vi "Usage Example.vi"() -> ()   [LabVIEW 2017, in "Client.lvlib" / "ParserSorter.lvlib"]
uses:
  ParserSorter.lvlib
  <vilib>/addons/database/Auxilliary.llb/DB Tools DataTypes.ctl
  SR Data.ctl
  AE Group.ctl
  SR Status.ctl
  SR Level.ctl
  SR Type.ctl
  <vilib>/addons/database/Connection.llb/DB Tools Open Connec (String).vi
  <vilib>/addons/database/NI_Database_API.lvlib
panel:
  out "Assigned":T1[](array[typedef])
  out "error out":errorcluster
  out "Unassigned":T1[](array[typedef])
  out "columns":string[](array[string])=["SR_NUMBER", "AE_GROUP", "SR_OWNER", "SR_SUMMARY", "SR_LAST_UPDATE_DATE", "FIRST_NAME", "LAST_NAME", "COMPANY", "SR_CREATION_DATE", "SR_TYPE", "SR_STATUS", "SERVICE_LEVEL", "CHANNEL", "DAYS_OPEN"]
  out "column information":T7(array[cluster])=[{"name"="SR_NUMBER", "database data type"=enum."String", "defined size"=64}, {"name"="AE_GROUP", "database data type"=enum."String", "defined size"=60}, {"name"="SR_OWNER", "database data type"=enum."String", "defined size"=721}, {"name"="SR_SUMMARY", "database data type"=enum."String", "defined size"=240}, {"name"="SR_LAST_UPDATE_DATE", "database data type"=enum."Date/Time", "defined size"=16}, {"name"="FIRST_NAME", "database data type"=enum."String", "defined size"=150}, {"name"="LAST_NAME", "database data type"=enum."String", "defined size"=150}, {"name"="COMPANY", "database data type"=enum."String", "defined size"=360}, {"name"="SR_CREATION_DATE", "database data type"=enum."Date/Time", "defined size"=16}, {"name"="SR_TYPE", "database data type"=enum."String", "defined size"=90}, {"name"="SR_STATUS", "database data type"=enum."String", "defined size"=90}, {"name"="SERVICE_LEVEL", "database data type"=enum."String", "defined size"=150}, {"name"="CHANNEL", "database data type"=enum."String", "defined size"=50}, {"name"="DAYS_OPEN", "database data type"=enum."Double (DBL)", "defined size"=8}]
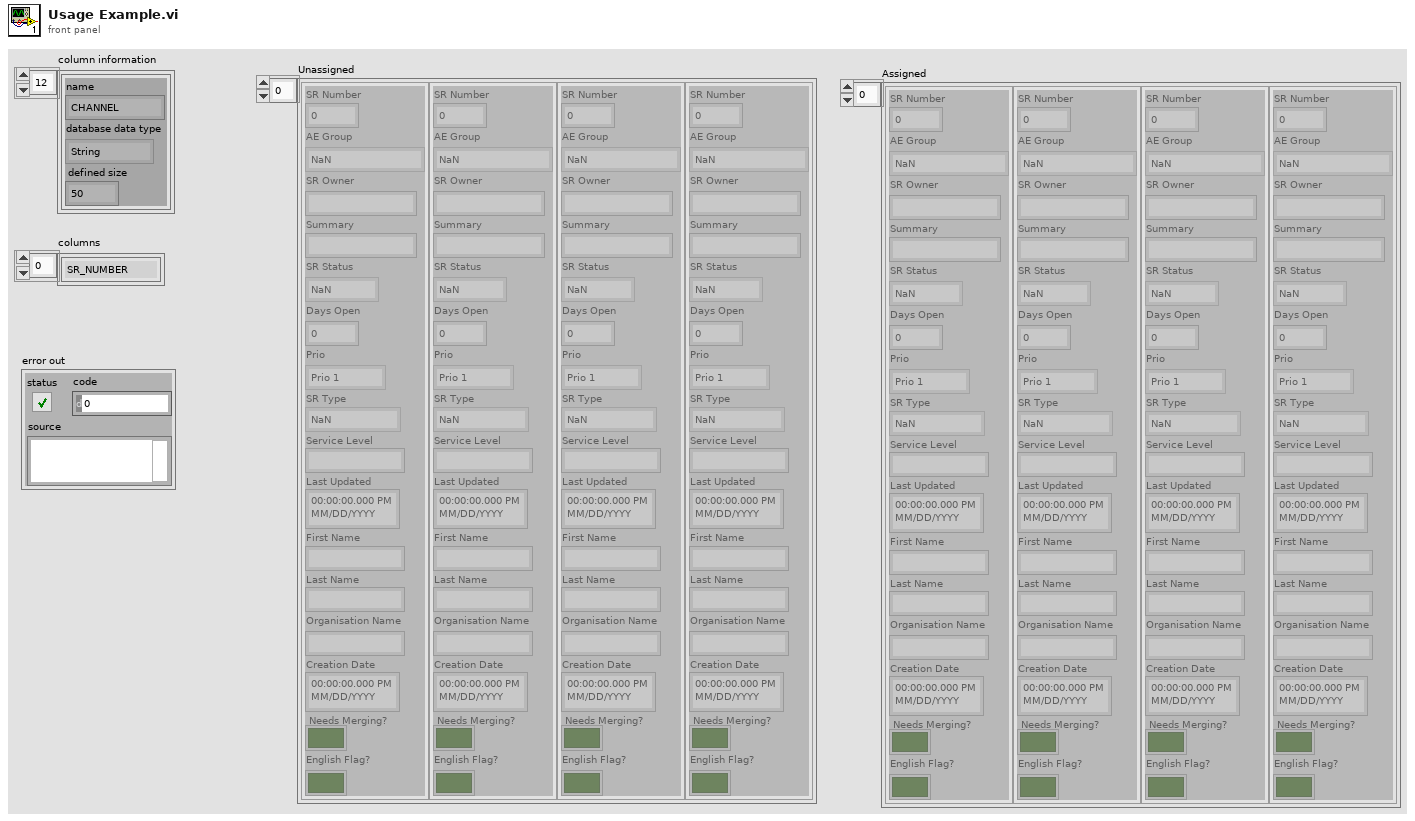
[diagram p1: front panel]
types:
  T1 = typedef "Client.lvlib/ParserSorter.lvlib/SR Data.ctl" = cluster{"SR Number":i64, "AE Group":T2, "SR Owner":string, "Summary":string, "SR Status":T3, "Days Open":dbl, "Prio":T4, "SR Type":T5, "Service Level":string, "Last Updated":timestamp, "First Name":string, "Last Name":string, "Organisation Name":string, "Creation Date":timestamp, "Needs Merging?":bool, "English Flag?":bool}
  T2 = typedef "Client.lvlib/ParserSorter.lvlib/AE Group.ctl" = enum32{"NaN", "AE-Germany", "AE-Poland", "AE-Switzerland", "AE-Czech Republic", "AE-Hungary", "AE-Romania", "AE-Slovakia", "AE-Slovenia"}
  T3 = typedef "Client.lvlib/ParserSorter.lvlib/SR Status.ctl" = enum32{"NaN", "Caller Abandoned", "Created in Error", "Declined to Purchase Support", "Expired", "Forum Resolved AE", "Forum Resolved Customer", "IN WORK", "IN WORK Collab with AES", "IN WORK Collab with PSE", "IN WORK Collab with SE", "IN WORK Escalation", "IN WORK Customer Added Note", "Open", "Potentially Resolved", "POC Resolved", "Resolved", "RMA Waiting on Customer", "RMA Open", "RMA In Progress", "RMA Closed - DOA", "RMA Closed", "RMA Approved for Return", "Project Complete", "Presumed Resolved", "IN WORK Wait on Customer"}
  T4 = typedef "Client.lvlib/ParserSorter.lvlib/SR Level.ctl" = enum16{"Prio 1", "Prio 2", "Prio 3", "Prio 4"}
  T5 = typedef "Client.lvlib/ParserSorter.lvlib/SR Type.ctl" = enum32{"NaN", "ATE Core Configurations (BYOATE)", "Activation", "BioBench", "CAN", "CM C Series", "Calibration", "Consulting Services", "CounterTimer", "DAQExpress", "DASYLab", "DIAdem", "DMM", "DSA HW", "Digital_IO", "FIRST (NIC Only)", "FieldBus", "FieldPoint", "Functional Savety", "GATI", "GPIB", "HMI and Industrial PCs", "HiQ", "HighSpeedDigital_IO", "IMAQ", "IOTech Vibration", "Industrial Communications", "InsightCM", "LV", "LV CD&Sim", "LV Comms", "LV Controls Add-Ons", "LV Embedded", "LV MathScript RT", "LV NXG", "LV NXT", "LVDSC", "LVFPGA", "LVPDA and LV Touch Panel", "LVRT", "LabWindows_CVI", "Lookout", "MATRIXx", "MStudioDotNet", "MStudioVisualBasic", "MStudioVisualC", "Measure (Legacy)", "Motion", "MultifunctionDAQ", "Multimedia Test HW/SW", "Multisim (EWB)", "NI Update Service", "OPC Servers", "Optical (OSI)", "PXI Controllers, Chassis, MXI", "PXI Timing and Sync", "Power Supplies and SMUs", "Powertrain Controls", "RAID", "RF", "RF Software", "RIO", "SC Express", "SCC", "SCXI", "SPEEDY-33 (Hyperception)", "STS", "ScopeDigitizers", "Serial", "Signal Sources", "SignalCondOther", "SignalExpress", "Software Defined Intruments", "Sound and Vibration SW", "Switch Executive", "Switches", "TestStand", "USRP", "Ultiboard (EWB)", "VBench", "VI Logger", "VXI_MXI", "VeriStand", "VisionSW", "VolumeLicenseMgr", "WSN", "Web UI Builder", "myRIO"}
  T6 = typedef "NI_Database_API.lvlib/DB Tools DataTypes.ctl" = enum16{"String", "Long (I32)", "Single (SGL)", "Double (DBL)", "Date/Time", "Binary"}
  T7 = cluster{"name":string, "database data type":T6, "defined size":i32}[]
  T8 = typedef "NI_Database_API.lvlib/Conn ObjectReference.ctl" = refnum<k1>
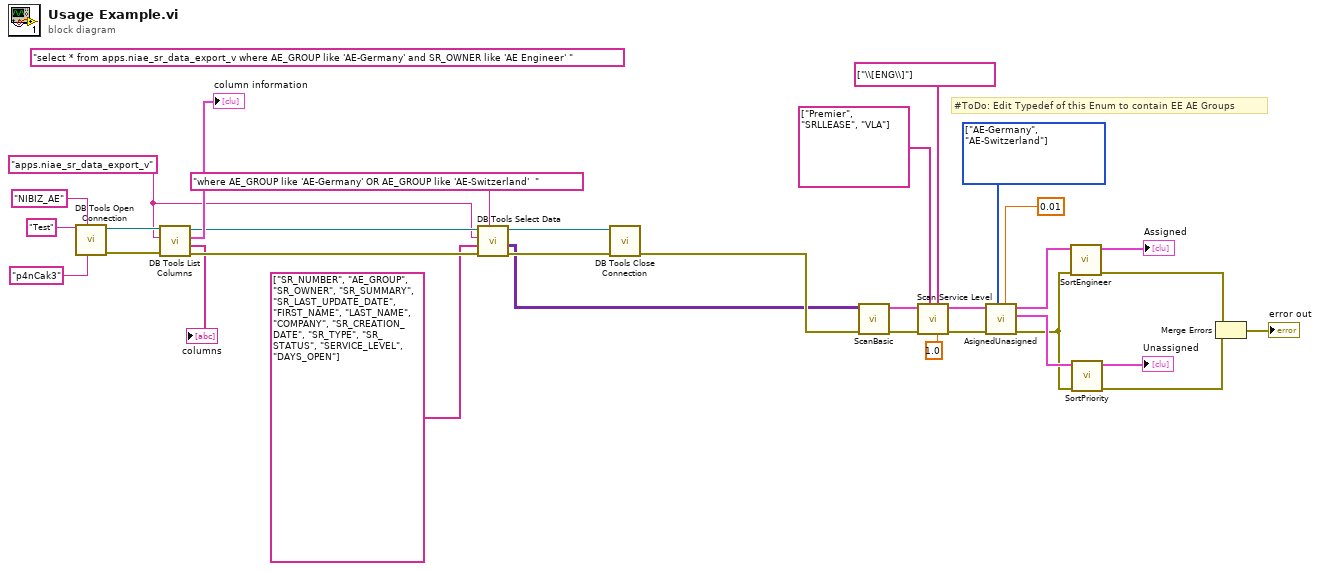
[diagram p0: block diagram]
diagram:
  w10 = "apps.niae_sr_data_export_v" ("table")
  (unwired) "select * from apps.niae_sr_data_export_v where AE_GROUP like 'AE-Germany' and SR_OWNER like 'AE Engineer' " ("SQL query")
  w19 = T2[] [enum."AE-Germany", enum."AE-Switzerland"] items=["NaN", "AE-Germany", "AE-Poland", "AE-Switzerland", "AE-Czech Republic", "AE-Hungary", "AE-Romania", "AE-Slovakia", "AE-Slovenia"] ("AE Groups")
  # "#ToDo: Edit Typedef of this Enum to contain EE AE Groups"
  n1 = call-poly <vilib>:"DB Tools Open Connection.vi"("password"="p4nCak3", "userID"="NIBIZ_AE", "connection information"="Test") -> ("error out"=w14:errorcluster, "connection reference"=w15:T8)  [unwired: 5 in]
  n2 = call <vilib>:"DB Tools List Columns.vi"("error in (no error)"=w14, "table"=w10, "connection reference"=w15) -> ("error out"=w11:errorcluster, "columns"=→"columns":string[], "column information"=→"column information":T7, "connection reference out"=w12:T8)  [unwired: 1 in]
  n3 = call <vilib>:"DB Tools Select Data.vi"("condition"="where AE_GROUP like 'AE-Germany' OR AE_GROUP like 'AE-Switzerland'  ", "error in (no error)"=w11, "columns"=string[] ["SR_NUMBER", "AE_GROUP", "SR_OWNER", "SR_SUMMARY", "SR_LAST_UPDATE_DATE", "FIRST_NAME", "LAST_NAME", "COMPANY", "SR_CREATION_DATE", "SR_TYPE", "SR_STATUS", "SERVICE_LEVEL", "DAYS_OPEN"] ("appended array"), "table"=w10, "connection reference"=w12) -> ("error out"=w6:errorcluster, "data"=w4:variant[][], "connection reference out"=w7:T8)  [unwired: 1 in]
  n4 = call <vilib>:"DB Tools Close Connection.vi"("error in (no error)"=w6, "connection reference"=w7) -> ("error out"=w33:errorcluster)  [unwired: 5 in]
  n5 = call "ScanBasic.vi"("error in (no error)"=w33, "data"=w4) -> ("error out"=w32:errorcluster, "Array"=w31:T1[])  [unwired: 8 in]
  n6 = call "Scan Service Level.vi"("Days Open Prio Threshold"=1.0 ("Days Open Treshhold"), "English Tags"=string[] ["\\[ENG\\]"], "Premier Levels Keywords"=string[] ["Premier", "SRLLEASE", "VLA"], "error in (no error)"=w32, "Array in"=w31) -> ("error out"=w23:errorcluster, "Array out"=w26:T1[])  [unwired: 5 in]
  n7 = call "AsignedUnasigned.vi"("Days Open Phone Treshhold"=0.01, "AE Groups"=w19, "error in (no error)"=w23, "All SR In"=w26) -> ("error out"=w24:errorcluster, "Unassigned"=w27:T1[], "Assigned Out"=w28:T1[])  [unwired: 5 in]
  n8 = call "SortEngineer.vi"("error in (no error)"=w24, "Array in"=w28) -> ("error out"=w3:errorcluster, "Array out"=→"Assigned":T1[])  [unwired: 8 in]
  n9 = call "SortPriority.vi"("error in (no error)"=w24, "Array in"=w27) -> ("error out"=w2:errorcluster, "Array out"=→"Unassigned":T1[])  [unwired: 8 in]
  n10 = Merge Errors(w3, w2) -> (→"error out":errorcluster)
